vi "Write Data.vi"(6 "Barcodes":string[](array[string]), 9 "Array":dbl[](array[numeric]), 10 "String":string) -> ()   [LabVIEW 2020]
uses:
  <vilib>/Utility/file.llb/Write Delimited Spreadsheet (string).vi
  <vilib>/Utility/file.llb/Write Delimited Spreadsheet (DBL).vi
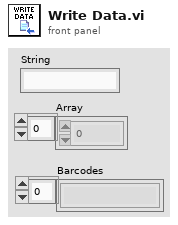
[diagram p1: front panel]
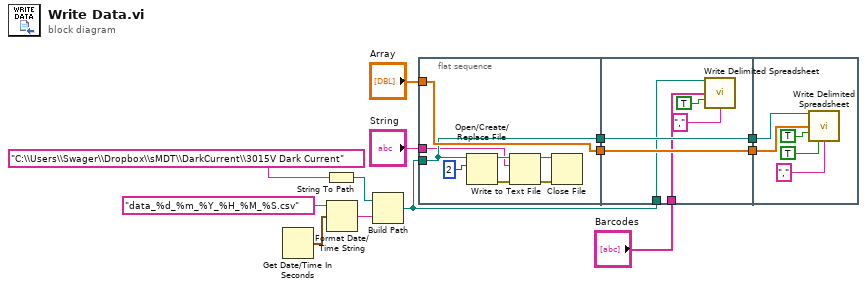
[diagram p0: block diagram]
diagram:
  n1 = Get Date/Time In Seconds() -> (seconds since 1Jan1904=w5:timestamp)
  n2 = String To Path(string="C:\\Users\\Swager\\Dropbox\\sMDT\\DarkCurrent\\3015V Dark Current") -> (path=w4:path)
  n3 = Format Date/Time String(time format string (%c)="data_%d_%m_%Y_%H_%M_%S.csv", seconds (now)=w5) -> (date/time string=w6:string)  [unwired: 1 in]
  n4 = Build Path(base path=w4, name or relative path=w6) -> (appended path=w1:path)
  n5 = flat-sequence {
    tunnel: w1 -> [w20]
    tunnel: [w20] -> w13
    tunnel: [w21] -> w12
    tunnel: "Array" -> [w21]
    tunnel: "String" -> [w17]
    tunnel: w13 -> [w27]
    tunnel: [w27] -> w11
    tunnel: w12 -> [w26]
    tunnel: [w26] -> w10
    tunnel: w1 -> [w25]
    tunnel: "Barcodes" -> [w24]
    tunnel: w11 -> [w30]
    tunnel: w10 -> [w29]
    frame #0 {
      n6 = Open/Create/Replace File(file path (use dialog)=w20, operation (0:open)=2) -> (refnum out=w18:refnum<file>, error out=w19:errorcluster)  [unwired: 4 in, 1 out]
      n7 = Write to Text File(file (use dialog)=w18, text=w17, error in=w19) -> (refnum out=w15:refnum<file>, error out=w16:errorcluster)  [unwired: 1 in, 1 out]
      n8 = Close File(refnum=w15, error in=w16) -> ()  [unwired: 2 out]
    }
    frame #1 {
      n9 = call-poly <vilib>:"Write Delimited Spreadsheet.vi"("file path (dialog if empty)"=w25, "1D data"=w24, "append to file? (new file:F)"=TRUE, "delimiter (\\t)"=",") -> ()  [unwired: 10 in, 2 out]
    }
    frame #2 {
      n10 = call-poly <vilib>:"Write Delimited Spreadsheet.vi"("file path (dialog if empty)"=w30, "1D data"=w29, "append to file? (new file:F)"=TRUE, "transpose? (no:F)"=TRUE, "delimiter (\\t)"=",") -> ()  [unwired: 9 in, 2 out]
    }
  }
